vi "Configure PRBS Waveform.vi"(4 "Amplitude Unit (0: Vpp)":u16(ring) items=["Vpp", "VRMS", "DBM"], 5 "Amplitude (0.1 Vpp)":dbl=0.1, 6 "Edge Time (8.4 ns)":dbl=8.4, 7 "Data Sequence (7: PN7)":u16(ring)=7 items=["PN7"=7, "PN9"=9, "PN11"=11, "PN15"=15, "PN20"=20, "PN23"=23, "PN3"=3, "PN4"=4, "PN5"=5, "PN6"=6, "PN8"=8, "PN10"=10, "PN12"=12, "PN13"=13, "PN14"=14, "PN16"=16, "PN17"=17, "PN18"=18, "PN19"=19, "PN21"=21, "PN22"=22, "PN24"=24, "PN25"=25, "PN26"=26, "PN27"=27, "PN28"=28, "PN29"=29, "PN30"=30, "PN31"=31, "PN32"=32], 8 "error in (no error)":errorcluster, 9 "Bit Rate (1000 bits/second)":dbl=1000.0, 10 "Channel (1: 1)":u16(ring)=1 items=["1"=1, "2"=2], 11 "VISA resource name":refnum<visa-resource-name>) -> (0 "error out":errorcluster, 3 "VISA resource name out":refnum<visa-resource-name>)   [LabVIEW 2020, in "Agilent 3352X Series.lvlib"]
doc: "Generates a PRBS waveform using polynomial PNx by a shift register of x bits, the output waveform will always begin with x sample periods of high output. \nSet bit rate, data sequence and transition edge time for PRBS function \nPRBS is Periodic Random Noise using Linear Feedback Shift Register (LFSR) methods selectable by the user (data sequence control). \n\n<b>Note</b>:\nSYNC Output may be active."
uses:
  Agilent 3352X Series.lvlib
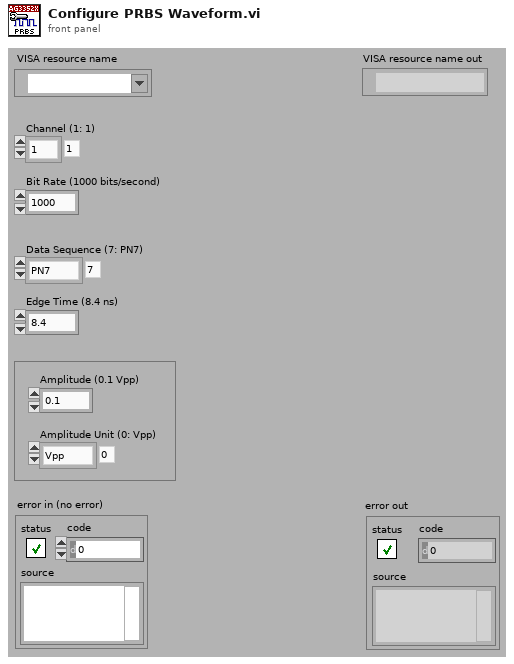
[diagram p1: front panel]
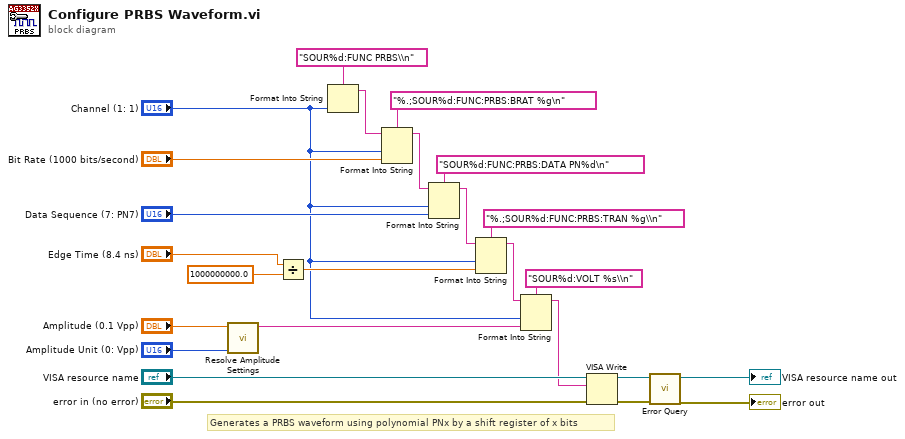
[diagram p0: block diagram]
diagram:
  # "Generates a PRBS waveform using polynomial PNx by a shift register of x bits"
  n1 = call "Resolve Amplitude Settings.vi"("Amplitude Unit (0: VPP)"="Amplitude Unit (0: Vpp)", "Amplitude (1 Vpp)"="Amplitude (0.1 Vpp)") -> ("Resulting String"=w8:string)  [unwired: 9 out]
  n2 = Divide(x="Edge Time (8.4 ns)", y=1000000000.0) -> (x/y=w10:dbl)
  n3 = Format Into String(format string="SOUR%d:FUNC PRBS\\n", "Channel (1: 1)") -> (resulting string=w3:string)  [unwired: 2 in, 1 out]
  n4 = Format Into String(format string="%.;SOUR%d:FUNC:PRBS:BRAT %g\n", initial string=w3, "Channel (1: 1)", "Bit Rate (1000 bits/second)") -> (resulting string=w23:string)  [unwired: 1 in, 1 out]
  n5 = Format Into String(format string="SOUR%d:FUNC:PRBS:DATA PN%d\n", initial string=w23, "Channel (1: 1)", "Data Sequence (7: PN7)") -> (resulting string=w20:string)  [unwired: 1 in, 1 out]
  n6 = Format Into String(format string="%.;SOUR%d:FUNC:PRBS:TRAN %g\\n", initial string=w20, "Channel (1: 1)", w10) -> (resulting string=w7:string)  [unwired: 1 in, 1 out]
  n7 = Format Into String(format string="SOUR%d:VOLT %s\\n", initial string=w7, "Channel (1: 1)", w8) -> (resulting string=w6:string)  [unwired: 1 in, 1 out]
  n8 = VISA Write(VISA resource name="VISA resource name", write buffer=w6, error in (no error)="error in (no error)") -> (VISA resource name out=w16:refnum<visa-resource-name>, error out=w15:errorcluster)  [unwired: 1 out]
  n9 = call "Error Query.vi"("error in (no error)"=w15, "VISA resource name"=w16) -> ("error out"=→"error out":errorcluster, "VISA resource name out"=→"VISA resource name out":refnum<visa-resource-name>)  [unwired: 8 out]
